vi "WS1050_Extract Data From Scope_ST_CLK.vi"(6 "95% Amp":dbl=0.95, 7 "60% Amp":dbl=0.6, 8 "error in (no error)":errorcluster, 11 "file path":path) -> (0 "error out":errorcluster, 1 "T1(us)":string, 2 "T2(us)":string, 3 "Amp(mv)":string, 5 "AMP(v)":dbl=1.1)   [LabVIEW 2012]
uses:
  <vilib>/Utility/file.llb/Read From Spreadsheet File (string).vi
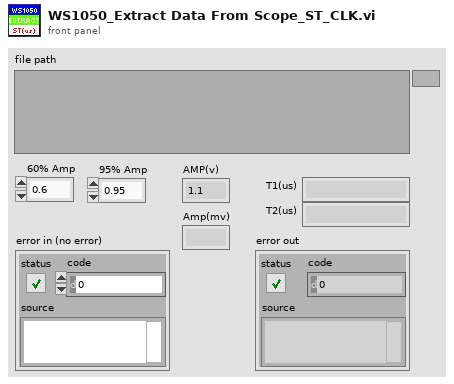
[diagram p1: front panel]
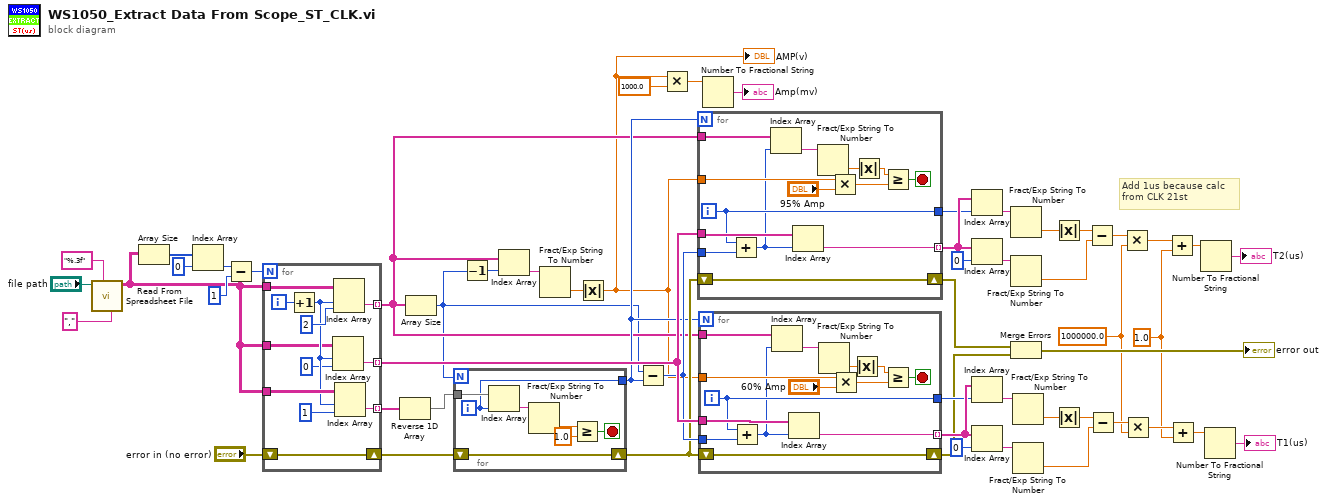
[diagram p0: block diagram]
diagram:
  w13 = 1.0 ("y")
  w14 = 1000000.0 ("y")
  # "Add 1us because calc \nfrom CLK 21st"
  n1 = call-poly <vilib>:"Read From Spreadsheet File.vi"("delimiter (\\t)"="," ("delimiter (\\t)"), "format (%s)"="%.3f" ("format (%.3f)"), "file path (dialog if empty)"="file path") -> ("all rows"=w43:string[][])  [unwired: 4 in, 4 out]
  n2 = Array Size(array=w43) -> (size(s)=w52:i32[])
  n3 = Index Array(array=w52, index=0) -> (element=w50:i32)
  n4 = Subtract(x=w50, y=1) -> (x-y=w49:i32)
  n5 = for {
    N: w49 -> [_]
    tunnel: w43 -> [w67]
    tunnel: [w64] -> w9 mode=indexing
    tunnel: w43 -> [w63]
    tunnel: [w61] -> w39 mode=indexing
    tunnel: w43 -> [w59]
    tunnel: [w57] -> w35 mode=indexing
    shift-right: [w56] -> w37
    shift-left: "error in (no error)" -> [w56]
    i -> [w65]
    n6 = Increment(x=w65) -> (x+1=w60:i32)
    n7 = Index Array(array=w59, index (row)=w60, index (col)=0 ("disabled index (col)")) -> (element=w57:string)
    n8 = Index Array(array=w67, index (row)=w60, index (col)=2 ("disabled index (col)")) -> (element=w64:string)
    n9 = Index Array(array=w63, index (row)=w60, index (col)=1 ("disabled index (col)")) -> (element=w61:string)
  }
  n10 = Reverse 1D Array(array=w39) -> (reversed array=w47:string[])
  n11 = Array Size(array=w9) -> (size(s)=w5:i32)
  n12 = for {
    N: w5 -> [_]
    tunnel: w47 -> [w74]
    tunnel: [w71] -> w12
    shift-right: [w69] -> w33
    shift-left: w37 -> [w69]
    i -> [w71]
    stop <- w72 stop-if-true
    n13 = Index Array(array=w74, index=w71) -> (element=w68:string)
    n14 = Fract/Exp String To Number(string=w68) -> (number=w70:dbl)  [unwired: 3 in, 1 out]
    n15 = Greater Or Equal?(x=w70, y=1.0) -> (x >= y?=w72:bool)
  }
  n16 = Decrement(x=w5) -> (x-1=w6:i32)
  n17 = Index Array(array=w9, index=w6) -> (element=w8:string)
  n18 = Fract/Exp String To Number(string=w8) -> (number=w7:dbl)  [unwired: 3 in, 1 out]
  n19 = Absolute Value(x=w7) -> (abs(x)=w2:dbl)
  "AMP(v)" <- w2
  n20 = Subtract(x=w5, y=w12) -> (x-y=w34:i32)
  n21 = Multiply(x=w2, y=1000.0) -> (x*y=w3:dbl)
  n22 = for {
    N: w12 -> [_]
    tunnel: w9 -> [w88]
    tunnel: w2 -> [w86]
    tunnel: w35 -> [w84]
    tunnel: [w83] -> w24 mode=indexing
    tunnel: [w81] -> w23
    tunnel: w34 -> [w82]
    shift-right: [w78] -> w31
    shift-left: w33 -> [w78]
    i -> [w81]
    stop <- w87 stop-if-true
    n23 = Add(x=w81, y=w82) -> (x+y=w80:i32)
    n24 = Index Array(array=w88, index=w80) -> (element=w75:string)
    n25 = Index Array(array=w84, index=w80) -> (element=w83:string)
    n26 = Fract/Exp String To Number(string=w75) -> (number=w77:dbl)  [unwired: 3 in, 1 out]
    n27 = Multiply(x=w86, y="95% Amp") -> (x*y=w85:dbl)
    n28 = Absolute Value(x=w77) -> (abs(x)=w76:dbl)
    n29 = Greater Or Equal?(x=w76, y=w85) -> (x >= y?=w87:bool)
  }
  n30 = for {
    N: w12 -> [_]
    tunnel: w9 -> [w102]
    tunnel: w2 -> [w100]
    tunnel: w35 -> [w98]
    tunnel: [w97] -> w42 mode=indexing
    tunnel: [w94] -> w41
    tunnel: w34 -> [w96]
    shift-right: [w91] -> w30
    shift-left: w33 -> [w91]
    i -> [w94]
    stop <- w101 stop-if-true
    n31 = Add(x=w94, y=w96) -> (x+y=w93:i32)
    n32 = Index Array(array=w102, index=w93) -> (element=w95:string)
    n33 = Index Array(array=w98, index=w93) -> (element=w97:string)
    n34 = Fract/Exp String To Number(string=w95) -> (number=w90:dbl)  [unwired: 3 in, 1 out]
    n35 = Multiply(x=w100, y="60% Amp") -> (x*y=w99:dbl)
    n36 = Absolute Value(x=w90) -> (abs(x)=w89:dbl)
    n37 = Greater Or Equal?(x=w89, y=w99) -> (x >= y?=w101:bool)
  }
  n38 = Number To Fractional String(number=w3) -> (F-format string=→"Amp(mv)":string)  [unwired: 3 in]
  n39 = Index Array(array=w24, index=w23) -> (element=w25:string)
  n40 = Index Array(array=w24, index=0) -> (element=w27:string)
  n41 = Index Array(array=w42, index=w41) -> (element=w46:string)
  n42 = Index Array(array=w42, index=0) -> (element=w44:string)
  n43 = Fract/Exp String To Number(string=w25) -> (number=w17:dbl)  [unwired: 3 in, 1 out]
  n44 = Fract/Exp String To Number(string=w27) -> (number=w11:dbl)  [unwired: 3 in, 1 out]
  n45 = Merge Errors(w31, w30) -> (→"error out":errorcluster)
  n46 = Fract/Exp String To Number(string=w46) -> (number=w15:dbl)  [unwired: 3 in, 1 out]
  n47 = Fract/Exp String To Number(string=w44) -> (number=w10:dbl)  [unwired: 3 in, 1 out]
  n48 = Absolute Value(x=w17) -> (abs(x)=w18:dbl)
  n49 = Absolute Value(x=w15) -> (abs(x)=w16:dbl)
  n50 = Subtract(x=w18, y=w11) -> (x-y=w28:dbl)
  n51 = Subtract(x=w16, y=w10) -> (x-y=w40:dbl)
  n52 = Multiply(x=w28, y=w14) -> (x*y=w19:dbl)
  n53 = Multiply(x=w40, y=w14) -> (x*y=w21:dbl)
  n54 = Add(x=w19, y=w13) -> (x+y=w20:dbl)
  n55 = Add(x=w21, y=w13) -> (x+y=w22:dbl)
  n56 = Number To Fractional String(number=w20) -> (F-format string=→"T2(us)":string)  [unwired: 3 in]
  n57 = Number To Fractional String(number=w22) -> (F-format string=→"T1(us)":string)  [unwired: 3 in]
